vi "Update PM File Name.vi"(8 "error in (no error)":errorcluster, 9 "All ROI In":T1[](array[typedef]), 10 "Old ROI Name":string, 11 "New Template Name":string) -> (0 "error out":errorcluster, 4 "All ROI Out":T1[](array[typedef]))   [LabVIEW 2019]
uses:
  Analysis/Controls/Parttern Match/Analysis_PatternMatch_Parameter.ctl
  Process/Controls/Process_Setting.ctl
  Analysis/Controls/Analysis_Setting.ctl
  Controls/Vision_DataEntry.ctl
  Analysis/Controls/V_Analysis_Type.ctl
  Ctrl/VisionProcessName.ctl
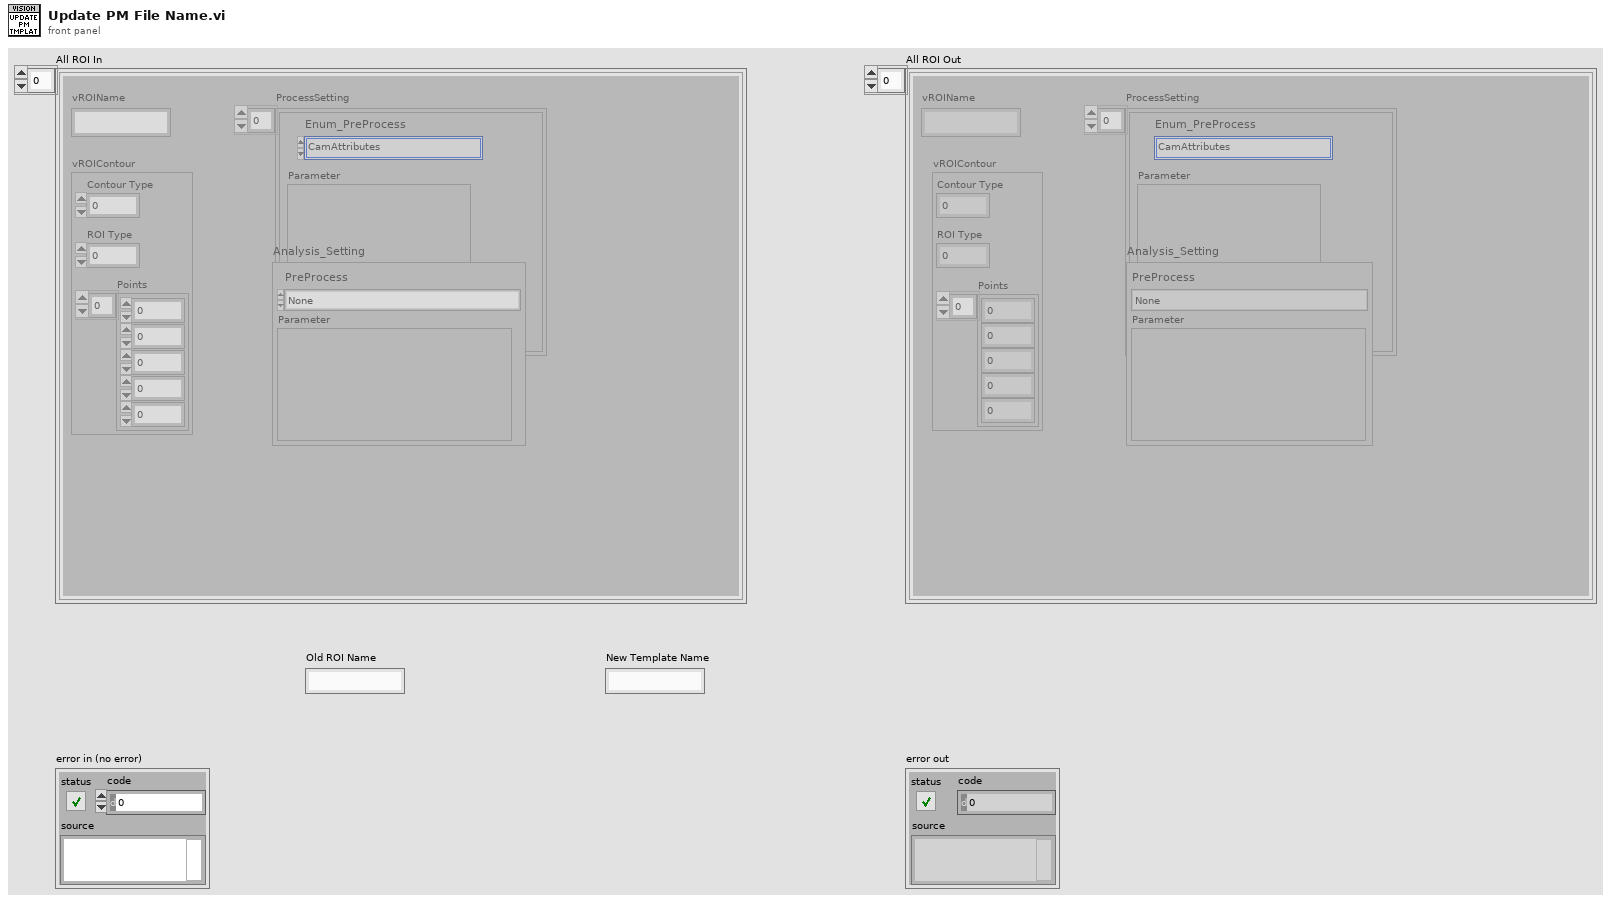
[diagram p1: front panel]
types:
  T1 = typedef "Vision_DataEntry.ctl" = cluster{"vROIName":string, "vROIContour":cluster{"Contour Type":u32, "ROI Type":u32, "Points":i32[]}, "ProcessSetting":T2[], "Analysis_Setting":T4}
  T2 = typedef "Process_Setting.ctl" = cluster{"Enum_PreProcess":T3, "Parameter":string}
  T3 = typedef "VisionProcessName.ctl" = enum16{"*CamParameter*", "CamAttributes", "*Preprocess*", "CG_Brightness", "C_Plane Extraction", "C_Threshold", "G_Lookup Table", "G_Threshold"}
  T4 = typedef "Analysis_Setting.ctl" = cluster{"PreProcess":T5, "Parameter":string}
  T5 = typedef "V_Analysis_Type.ctl" = enum16{"None", "C_Color Pattern Matching", "G_PatternMatching", "G_ShapeDectect", "G_GeometricMatch", "B_Area Check"}
  T6 = typedef "Analysis_PatternMatch_Parameter.ctl" = cluster{"Algorithm":i32, "Match Parameters":cluster{"Number of Matches Requested":i32, "Minimum Match Score":sgl, "Angle Ranges":cluster{"Start Angle":sgl, "End Angle":sgl}[]}, "ROI Descriptor":T7, "Advanced Options":cluster{"Item":u16, "Value":dbl}[], "Template path":string, "XOffset":i32, "YOffset":i32}
  T7 = typedef "ROI Descriptor" = cluster{"Global Rectangle":i32[], "Contours":cluster{"ID":enum32{"External", "Internal"}, "Type":u32, "Coordinates":i32[]}[]}
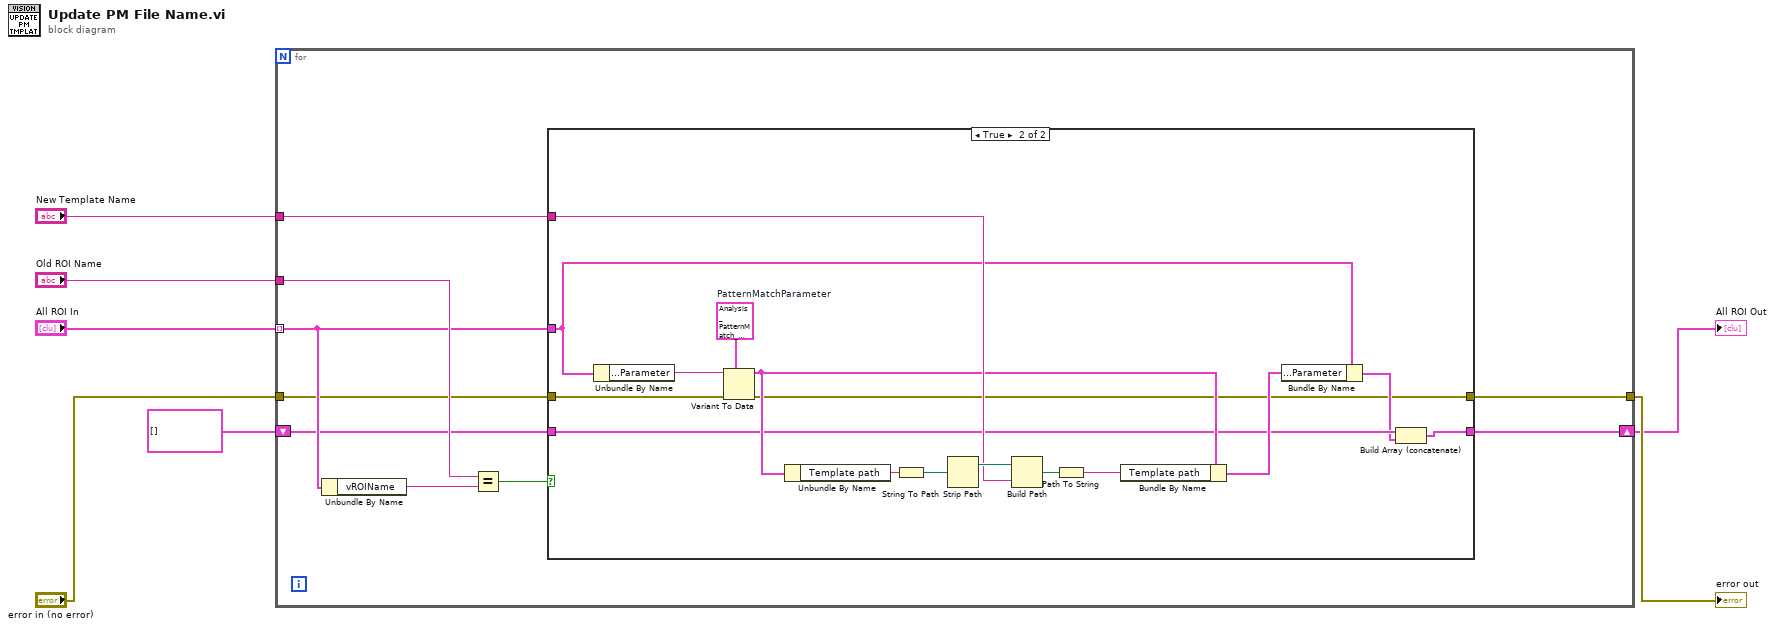
[diagram p0: block diagram]
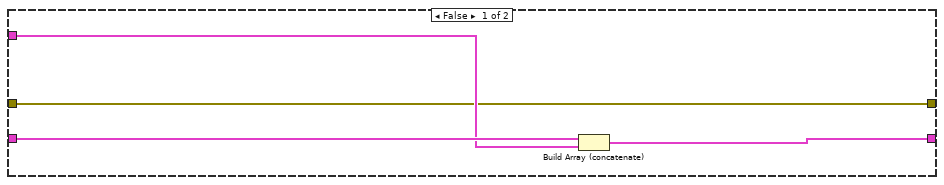
[diagram p2: hidden frame]
diagram:
  n1 = for {
    tunnel: "All ROI In" -> [w13] mode=indexing
    tunnel: "Old ROI Name" -> [w15]
    shift-right: [w11] -> w1
    shift-left: T1[] [] -> [w12]
    tunnel: [w10] -> w5
    tunnel: "error in (no error)" -> [w9]
    tunnel: "New Template Name" -> [w8]
    n2 = Unbundle By Name(w13) -> ("vROIName"=w16:string)
    n3 = Equal?(x=w15, y=w16) -> (x = y?=w14:bool)
    n4 = case shown="True" w14 {
      tunnel: w13 -> [w19 w27]
      tunnel: w8 -> [_ w31]
      tunnel: w12 -> [w20 w25]
      tunnel: [w18 w23] -> w11
      tunnel: [w17 w22] -> w10
      tunnel: w9 -> [w17 w21]
      frame False {
        n5 = Build Array (concatenate)(w20, w19) -> (w18:T1[])
      }
      frame True {
        w35 = T6 {"Algorithm"=2, "Match Parameters"={"Number of Matches Requested"=1, "Minimum Match Score"=750.0, "Angle Ranges"=[]}, "ROI Descriptor"={"Global Rectangle"=[], "Contours"=[]}, "Advanced Options"=[{"Item"=1, "Value"=1.0}, {"Item"=103, "Value"=1.0}], "Template path"="", "XOffset"=0, "YOffset"=0}  # PatternMatchParameter
        n6 = Unbundle By Name(w27) -> ("Analysis_Setting.Parameter"=w36:string)
        n7 = Variant To Data(error in=w21, type=w35, Variant=w36) -> (data=w29:T6, error out=w22:errorcluster)
        n8 = Unbundle By Name(w29) -> ("Template path"=w34:string)
        n9 = String To Path(string=w34) -> (path=w33:path)
        n10 = Strip Path(path=w33) -> (stripped path=w32:path)  [unwired: 1 out]
        n11 = Build Path(base path=w32, name or relative path=w31) -> (appended path=w30:path)
        n12 = Path To String(path=w30) -> (string=w28:string)
        n13 = Bundle By Name(cluster=w29, "Template path"=w28) -> (w26:T6)
        n14 = Bundle By Name(cluster=w27, "Analysis_Setting.Parameter"=w26) -> (w24:T1)
        n15 = Build Array (concatenate)(w25, w24) -> (w23:T1[])
      }
    }
  }
  "error out" <- w5
  "All ROI Out" <- w1
